vi "Module Name--constant.vi"() -> (3 "Module Name":string)   [LabVIEW 2025, in "Logger.lvlib"]
doc: "Return the name of the module that owns this VI. \n_____\nBased on DQMH Project Template 4.0.0.47.\n_____\nBased on DQMH Dev Tools: Project Template 7.1.0.1503."
uses:
  Logger.lvlib
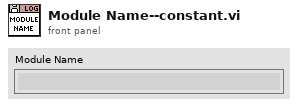
[diagram p1: front panel]
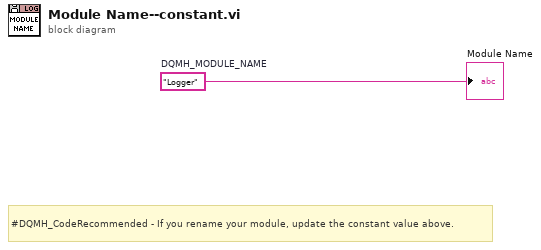
[diagram p0: block diagram]
diagram:
  w1 = "Logger"  # DQMH_MODULE_NAME
  # "#DQMH_CodeRecommended - If you rename your module, update the constant value above."
  "Module Name" <- w1
